vi "CODCr测量状态.vi"() -> ()   [LabVIEW 2016, in "CODCr库.lvlib"]
panel:
  out "工作状态":T1(ring)
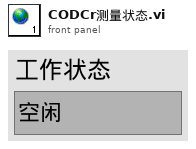
[diagram p1: front panel]
types:
  T1 = enum16{"空闲", "水样测试", "标样核查", "零点核查", "跨度核查", "空白测试", "平行样测试", "加标回收", "空白校准", "标样校准", "初始化（清洗）"}
diagram:
